vi "ElementWiseAbs.vi"(11 "Array [in]":dbl[](array[numeric])) -> (3 "Array[out]":dbl[](array[numeric]))   [LabVIEW 2012]
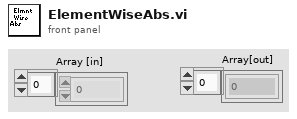
[diagram p1: front panel]
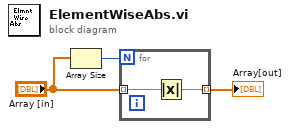
[diagram p0: block diagram]
diagram:
  n1 = Array Size(array="Array [in]") -> (size(s)=w3:i32)
  n2 = for {
    N: w3 -> [_]
    tunnel: "Array [in]" -> [w5] mode=indexing
    tunnel: [w4] -> w1 mode=indexing
    n3 = Absolute Value(x=w5) -> (abs(x)=w4:dbl)
  }
  "Array[out]" <- w1
